vi "getStateName.vi"(9 "error in (no error)":errorcluster, 11 "shuttingDown in":refnum<class "shuttingDown.lvclass">) -> (1 "error out":errorcluster, 2 "State Name":string, 3 "shuttingDown out":refnum<class "shuttingDown.lvclass">)   [LabVIEW 2020, in "eos.lvlib" / "shuttingDown.lvclass"]
uses:
  shuttingDown.lvclass
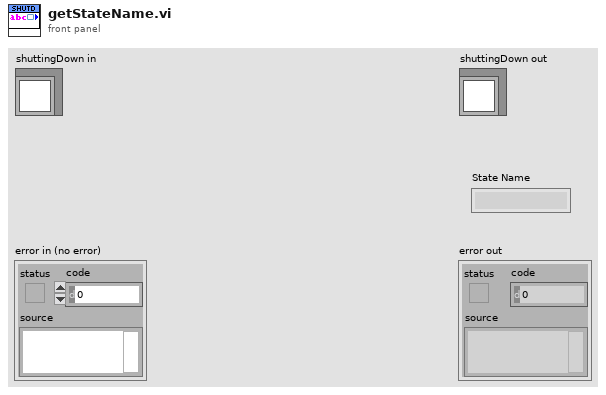
[diagram p1: front panel]
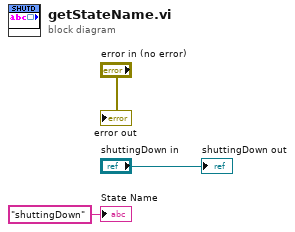
[diagram p0: block diagram]
diagram:
  "error out" <- "error in (no error)"
  "shuttingDown out" <- "shuttingDown in"
  "State Name" <- "shuttingDown" ("State Name")
